vi "Get Registry Data.vi"(8 "error in (no error)":errorcluster, 11 "Registry in":refnum<class "Registry.lvclass">) -> (0 "error out":errorcluster, 2 "Registry Data":variant)   [LabVIEW 2020, in "BCI-1553 API.lvlib" / "Registry.lvlib" / "Registry.lvclass"]
doc: "Retrieves the variant used for storing the Key/Value pairs in the Registry."
uses:
  Registry.lvclass
  Registry.lvclass/Registry.ctl
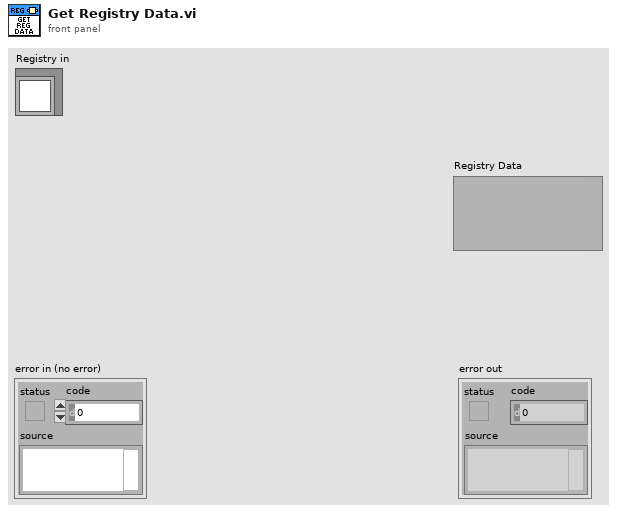
[diagram p1: front panel]
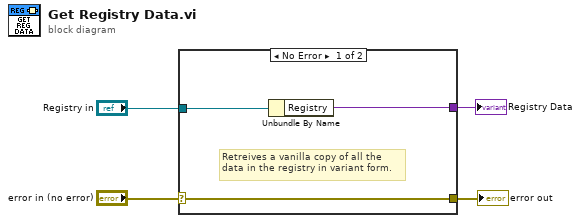
[diagram p0: block diagram]
diagram:
  n1 = case shown="No Error" "error in (no error)" {
    selector: "error in (no error)" -> [w7 w8]
    tunnel: [w7 w8] -> w3
    tunnel: "Registry in" -> [w6 _]
    tunnel: [w5 _] -> w1
    frame No Error {
      # "Retreives a vanilla copy of all the\ndata in the registry in variant form."
      n2 = Unbundle By Name(w6) -> ("Registry"=w5:variant)
    }
    frame Error {
    }
  }
  "error out" <- w3
  "Registry Data" <- w1
